vi "Write (I16).vi"(0 "disk streaming in":refnum<class "Disk Streaming.lvclass">, 1 "sample data":i16[](array[numeric]), 3 "elements remaining":u32, 5 "error in (no error)":errorcluster) -> (13 "finished":bool, 14 "disk streaming out":refnum<class "Disk Streaming.lvclass">, 18 "number of pending writes":u32, 19 "error out":errorcluster)   [LabVIEW 2021, in "Disk Streaming.lvclass"]
doc: "Writes data to a file in the streaming process controlled by a disk streaming instance and generates status information. For more information about the disk streaming instance refer to the <B>Open.vi</B> context help.\n\nUse this VI when streaming to disk using the TDMS Advanced Synchronous I/O functions or the TDMS Advanced Asynchronous I/O functions (the disk streaming instance was created by the <B>Open.vi</B> with the <B>disk read (F) / write (T)</B> input set to true and the <B>I/O mode</B> input set to \"Synchronous\" or \"Asynchronous\"). The streaming process requires the execution of the following sequence in a loop:\n1. Use the <B>Get Next Transfer Size.vi</B> to obtain the number of elements to transfer in the current iteration. If this VI returns zero, then the streaming is complete.\n2. Call the Read FIFO method on the Target to Host FIFO transferring the data from the FPGA Target to read the data to write to the file. Use the value returned by the <B>Get Next Transfer Size.vi</B> on the \"Number of Elements\" input of the FIFO method.\n3. Call this VI using the outputs returned by the FIFO method.\n\nInputs:\n\n<B>disk streaming in</B>: Disk streaming instance input.\n\n<B>sample data</B>: Array of I16s to write to the file. Wire the \"Data\" output of the FIFO method reading the Target to Host FIFO to this input.\n\n<B>elements remaining</B>: Set this input to the number of additional elements remaining in the host DMA buffer that are available for reading. This input is used only in the calculation of the Host DMA buffer utilization status. Wire the \"Elements Remaining\" output of the FIFO method reading the Target to Host FIFO to this input.\n\nOutputs:\n\n<B>disk streaming out</B>: Disk streaming instance output. Pass this output to the other Disk Streaming VIs to perform the streaming.\n\n<B>number of pending writes</B>: The number of asynchronous writes that are currently running in the background. Use the <B>Get Status.vi</B> to obtain additional status information.\n\n<B>finished</B>: Indicates whether the streaming is finished."
uses:
  Disk Streaming.lvclass
  Disk Streaming.lvclass/Disk Streaming.ctl
  <vilib>/Utility/error.llb/Error Cluster From Error Code.vi
  <vilib>/ErrorRing/Error Ring.xnode
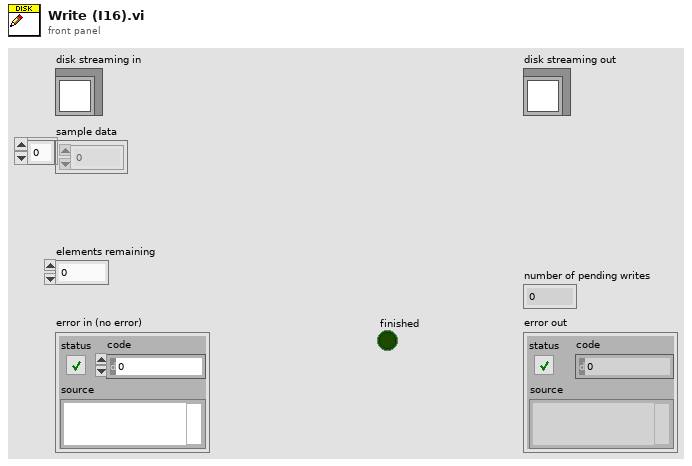
[diagram p1: front panel]
types:
  T1 = typedef "Disk Streaming.lvclass/Data.ctl" = cluster{"tdms file":refnum<k34>, "group name":string, "channel name":string, "max operations":u32, "timeout (s)":dbl, "data type size (bytes)":u64, "writing":bool, "I/O mode":T2, "# of blocks":u32, "block size divisor (bytes)":u32, "file position (elements)":u64, "file size (elements)":i64, "file size (samples)":i64, "block size (elements)":u64, "block size (samples)":u64, "quantum size (elements)":u64, "quantum size (samples)":u64, "samples remaining":i64, "elements transferred":u64, "finished":bool, "preview size":i32, "preview quantum size (elements)":u64, "preview quantum size (samples)":u64, "DMA buffer size (elements)":u32, "pending block sizes (bytes)":u64[]}
  T2 = typedef "Disk Streaming.lvclass/IO mode.ctl" = enum16{"Synchronous", "Asynchronous", "Data Reference"}
  T3 = typedef "Disk Streaming.lvclass/Status.ctl" = cluster{"finished":bool, "Host DMA buffer size (bytes)":u64, "Host DMA buffer utilization (bytes)":u64, "Disk maximum async operations":u32, "Disk pending async operations":u32, "preview data":i16[]}
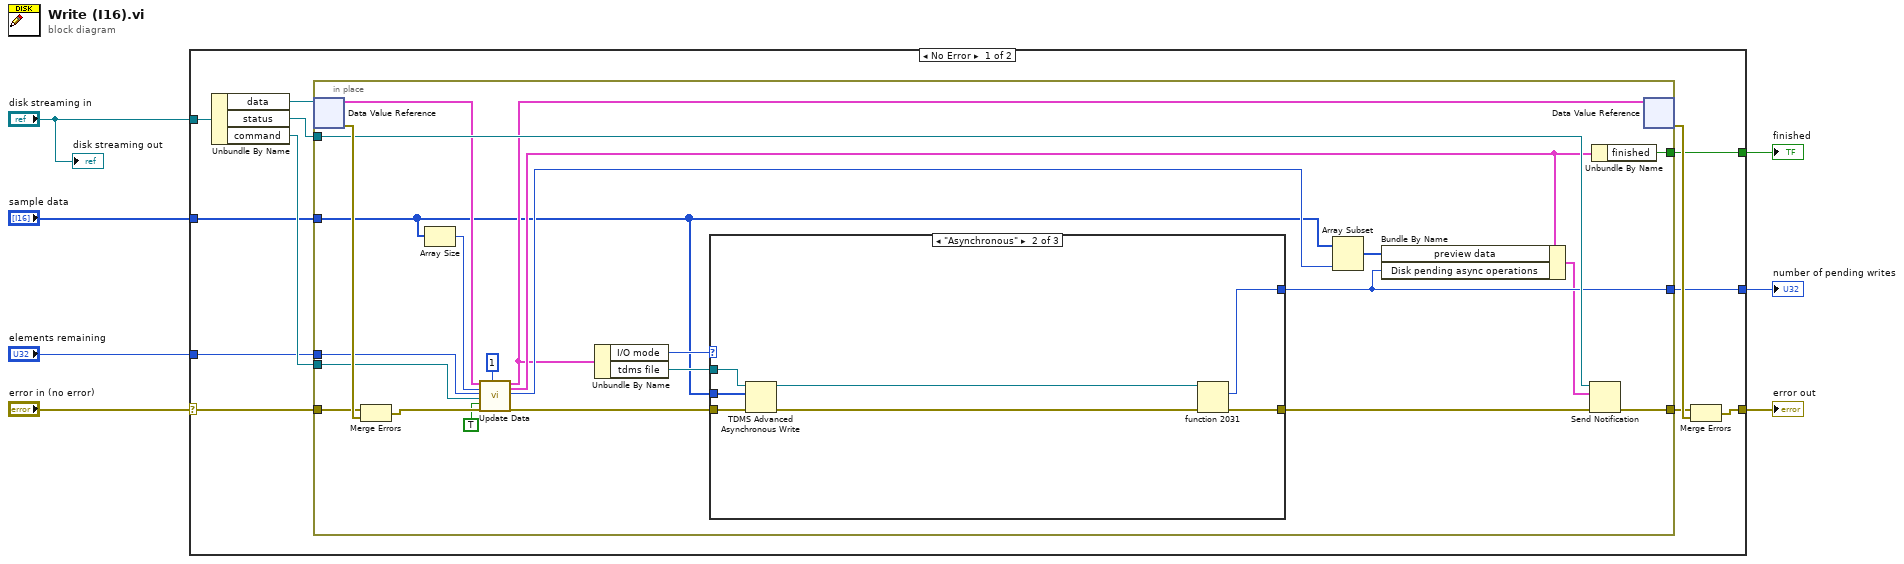
[diagram p0: block diagram]
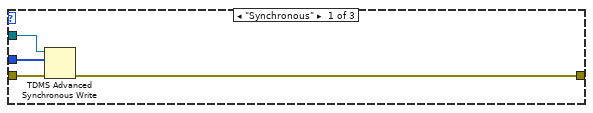
[diagram p2: hidden frame]
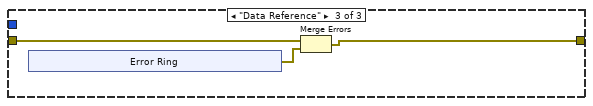
[diagram p3: hidden frame]
diagram:
  n1 = case shown="No Error" "error in (no error)" {
    selector: "error in (no error)" -> [w17 w62]
    tunnel: [w16 w62] -> w6
    tunnel: "sample data" -> [w11 _]
    tunnel: [w14 _] -> w4
    tunnel: "elements remaining" -> [w10 _]
    tunnel: "disk streaming in" -> [w13 _]
    tunnel: [w8 _] -> w1
    frame No Error {
      n2 = Unbundle By Name(w13) -> ("data"=w12:refnum<data-value>, "status"=w9:refnum<notifier>, "command"=w19:refnum<notifier>)
      n3 = in-place {
        in-place-border: w17 -> [w38]
        in-place-border: [w29] -> w15
        in-place-border: [w37] -> w14
        in-place-border: w19 -> [w33]
        in-place-border: w11 -> [w20]
        in-place-border: w10 -> [w34]
        in-place-border: w9 -> [w40]
        in-place-border: [w27] -> w8
        n4 = in-place-dvr #1(w12) -> (w23:T1, w41:errorcluster)
        n5 = Merge Errors(w38, w41) -> (w39:errorcluster)
        n6 = Array Size(array=w20) -> (size(s)=w35:i32)
        n7 = call "Update Data.vi"("data in"=w23, "block size (elements)"=w35, "(empty) elements remaining"=w34, "command"=w33, "writing?"=TRUE, "error in (no error)"=w39, "pending blocks in host buffer"=1) -> ("data out"=w22:T1, "status"=w25:T3, "preview size (elements)"=w42:i32, "error out"=w31:errorcluster)  [unwired: 7 in, 2 out]
        n8 = Unbundle By Name(w22) -> ("I/O mode"=w21:T2, "tdms file"=w28:refnum<k34>)
        n9 = case shown="\"Asynchronous\"" w21 {
          tunnel: [_ w51 _] -> w37
          tunnel: w31 -> [w46 w50 w55]
          tunnel: [w43 w49 w54] -> w30
          tunnel: w28 -> [w45 w48 _]
          tunnel: w20 -> [w44 w47 _]
          frame "Synchronous" {
            n10 = TDMS Advanced Synchronous Write(8:w46, 10:w44, 11:w45) -> (0:w43:errorcluster)  [unwired: 1 out]
          }
          frame "Asynchronous" {
            n11 = TDMS Advanced Asynchronous Write(8:w50, 10:w47, 11:w48) -> (0:w53:errorcluster, 3:w52:refnum<k34>)
            n12 = fn#2031(8:w53, 11:w52) -> (0:w49:errorcluster, 2:w51:u32)  [unwired: 1 out]
          }
          frame "Data Reference" {
            n13 = xnode "Error Ring"() -> ("error out"=w56:errorcluster)
            n14 = Merge Errors(w55, w56) -> (w54:errorcluster)
          }
        }
        n15 = Array Subset(array=w20, length=w42) -> (w26:i16[])  [unwired: 1 in]
        n16 = Bundle By Name(cluster=w25, "preview data"=w26, "Disk pending async operations"=w37) -> (w36:T3)
        n17 = Send Notification(notification=w36, notifier=w40, error in (no error)=w30) -> (error out=w29:errorcluster)  [unwired: 1 out]
        n18 = Unbundle By Name(w25) -> ("finished"=w27:bool)
        n19 = in-place-dvr #1(w22) -> (w18:errorcluster)  [unwired: 1 out]
      }
      n20 = Merge Errors(w15, w18) -> (w16:errorcluster)
    }
    frame Error {
    }
  }
  "error out" <- w6
  "number of pending writes" <- w4
  "finished" <- w1
  "disk streaming out" <- "disk streaming in"
